vi "Delete Duplicate Array Items.vi"(11 "Files":path[](array[path])) -> (3 "Files":path[](array[path]))   [LabVIEW 2023]
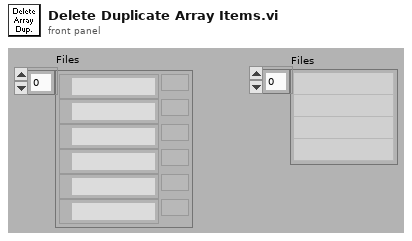
[diagram p1: front panel]
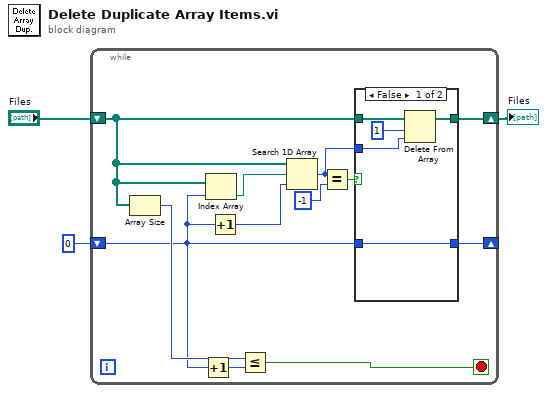
[diagram p0: block diagram]
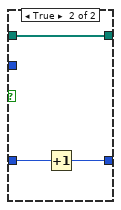
[diagram p2: hidden frame]
diagram:
  n1 = while {
    shift-right: [w10] -> w2
    shift-left: "Files" -> [w11]
    shift-right: [w5] -> _
    shift-left: 0 ("size(s)") -> [w6]
    stop <- w14 stop-if-true
    n2 = Array Size(array=w11) -> (size(s)=w15:i32)
    n3 = Increment(x=w6) -> (x+1=w7:i32)
    n4 = Index Array(array=w11, index=w6) -> (element=w13:path)
    n5 = Increment(x=w6) -> (x+1=w12:i32)
    n6 = Less Or Equal?(x=w15, y=w7) -> (x <= y?=w14:bool)
    n7 = Search 1D Array(1D array=w11, element=w13, start index (0)=w12) -> (index of element=w4:i32)
    n8 = Equal?(x=w4, y=-1) -> (x = y?=w8:bool)
    n9 = case shown="False" w8 {
      tunnel: w11 -> [w20 w23]
      tunnel: [w18 w23] -> w10
      tunnel: w6 -> [w17 w22]
      tunnel: [w17 w21] -> w5
      tunnel: w4 -> [w16 _]
      frame False {
        n10 = Delete From Array(array=w20, length=1, index=w16) -> (array with subset deleted=w18:path[])  [unwired: 1 out]
      }
      frame True {
        n11 = Increment(x=w22) -> (x+1=w21:i32)
      }
    }
  }
  "Files" <- w2
